vi "Commit Properties for Session.vi"(0 "session in":refnum<k21>, 11 "error in (no error)":errorcluster) -> (4 "session out":refnum<k21>, 15 "error out":errorcluster)   [LabVIEW 2020, in "SLSC.lvlib"]
doc: "Commits all device and physical channel properties with pending changes to hardware, for all devices and physical channels used by the session. If you set a property multiple times between commits, only the last value will be committed."
uses:
  <vilib>/SLSC/SLSC.lvlib
  nislsclvapi.dll
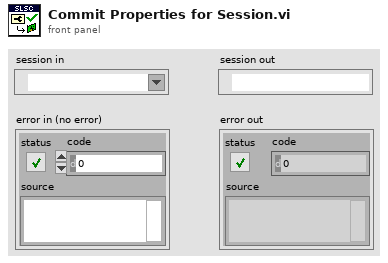
[diagram p1: front panel]
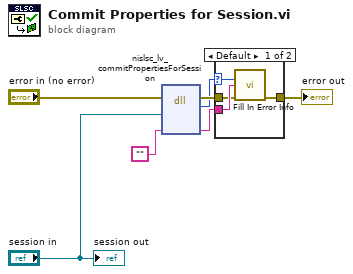
[diagram p0: block diagram]
diagram:
  n1 = dll-call lib="nislsclvapi.*" fn="nislsc_lv_commitPropertiesForSession"(error in="error in (no error)", "session"="session in", "extendedErrorInfo"="") -> (error out=w5:errorcluster, "return type"=w4:i32, "extendedErrorInfo"=w6:string)  [unwired: 5 in, 1 out]
  n2 = case shown="Default" w4 {
    selector: w4 -> [w11 _]
    tunnel: w6 -> [w10 _]
    tunnel: w5 -> [w9 w12]
    tunnel: [w8 w12] -> w3
    frame Default {
      n3 = call <vilib>:"Fill In Error Info.vi"("status code"=w11, "extended error info"=w10, "error in"=w9) -> ("error out"=w8:errorcluster)  [unwired: 12 in]
    }
    frame 0 {
    }
  }
  "error out" <- w3
  "session out" <- "session in"
